vi "Example Unbundler 1.vi"() -> ()   [LabVIEW 2014]
panel:
  out "ind3":string[](array[string])
  out "ind1":string
  out "ind2":i32
  out "Error Out":errorcluster
  in  "Error In":errorcluster
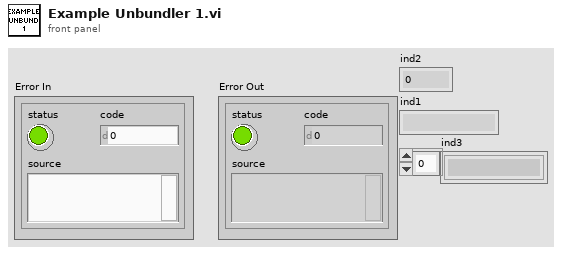
[diagram p1: front panel]
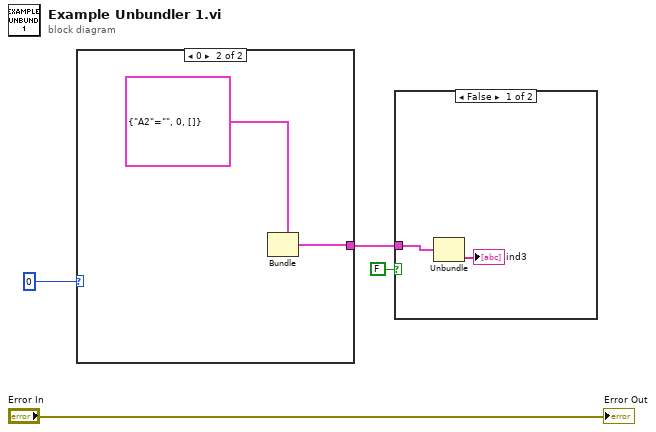
[diagram p0: block diagram]
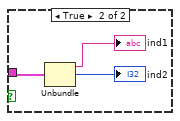
[diagram p2: hidden frame]
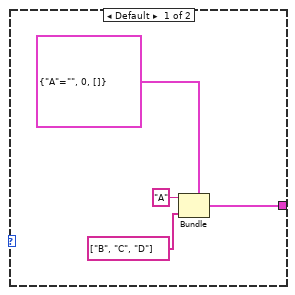
[diagram p3: hidden frame]
diagram:
  n1 = case shown="0" 0 {
    tunnel: [w5 w9] -> w1
    frame Default {
      n2 = Bundle(cluster=cluster{"A":string, i32, string[]} {"A"="", 0, []}, "A"="A", string[] ["B", "C", "D"]) -> (w5:cluster{"A":string, i32, string[]})  [unwired: 1 in]
    }
    frame 0 {
      n3 = Bundle(cluster=cluster{"A2":string, i32, string[]} {"A2"="", 0, []}) -> (w9:cluster{"A2":string, i32, string[]})  [unwired: 3 in]
    }
  }
  n4 = case shown="False" FALSE {
    tunnel: w1 -> [w12 w15]
    frame False {
      n5 = Unbundle(w12) -> (→"ind3":string[])  [unwired: 2 out]
    }
    frame True {
      n6 = Unbundle(w15) -> ("A2"=→"ind1":string, →"ind2":i32)  [unwired: 1 out]
    }
  }
  "Error Out" <- "Error In"
